vi "Load EEPROM Data FTS Main.vi"(8 "error in (no error)":errorcluster) -> (0 "error out":errorcluster, 3 "EEPROM data":u8[][](array[numeric]) format="%02x")   [LabVIEW 2015]
uses:
  <vilib>/addons/_office/excel.llb/Excel Get Data ([str]).vi
  <vilib>/Utility/NIReport.llb/NI_report.lvclass
  <vilib>/addons/_office/NI_ReportGenerationToolkit.lvlib
  <vilib>/Utility/NIReport.llb/Excel/NI_Excel.lvclass
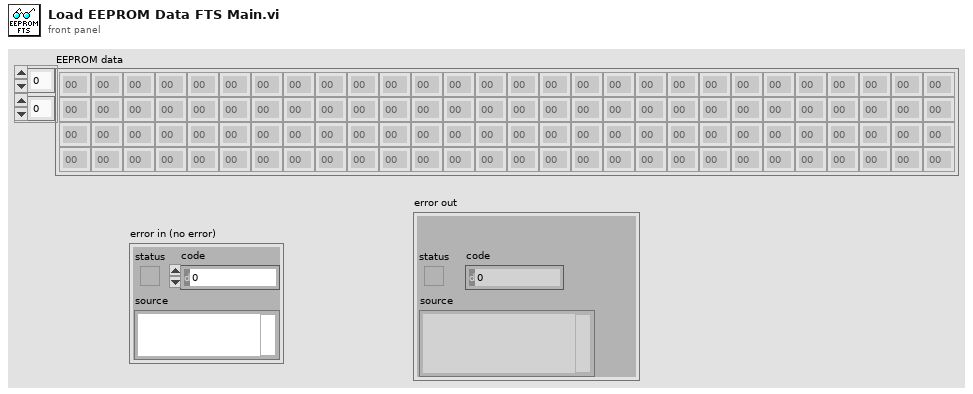
[diagram p1: front panel]
types:
  T1 = enum16{"maximized", "minimized", "normal", "no change"}
  T2 = enum16{"Standard Report", "HTML", "Word", "Excel"}
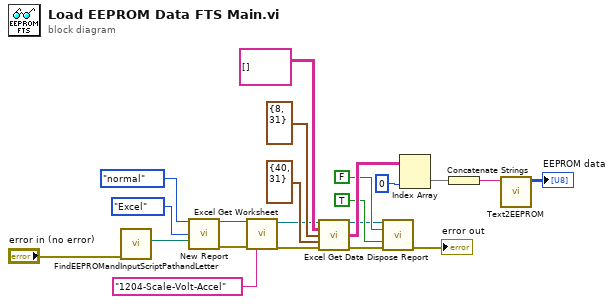
[diagram p0: block diagram]
diagram:
  n1 = call "FindEEPROMandInputScriptPathandLetter.vi"("Error In"="error in (no error)") -> ("Engr Result Path"=w22:path)  [unwired: 6 in, 2 out]
  n2 = call <vilib>:"New Report.vi"("window state (normal)"=T1."normal", "report type"=T2."Excel", "template (empty)"=w22) -> ("report out"=w19:refnum<class "NI_report.lvclass">, "error out"=w18:errorcluster)  [unwired: 11 in]
  n3 = call <vilib>:"Excel Get Worksheet.vi"("report in"=w19, "error in (no error)"=w18, "name (\"\")"="1204-Scale-Volt-Accel" ("name (\"\")")) -> ("report out"=w4:refnum<class "NI_report.lvclass">, "error out"=w6:errorcluster)  [unwired: 11 in]
  n4 = call-poly <vilib>:"Excel Get Data.vi"("report in"=w4, "data type"=string[][] [], "start (-1, -1)"=cluster{"row":i32, "column":i32} {"row"=8, "column"=31}, "end (-1, -1)"=cluster{"row":i32, "column":i32} {"row"=40, "column"=31}, "error in (no error)"=w6) -> ("report out"=w3:refnum<class "NI_report.lvclass">, "data"=w14:string[][], "error out"=w2:errorcluster)  [unwired: 8 in]
  n5 = call-dynamic "Dispose Report.vi"("report in"=w3, "wait until printing completed? (T)"=FALSE, "save changes? (F)"=TRUE, "error in (no error)"=w2) -> ("error out"=→"error out":errorcluster)  [unwired: 11 in]
  n6 = Index Array(array=w14, index (col)=0 ("disabled index (col)")) -> (element=w11:string[])  [unwired: 1 in]
  n7 = Concatenate Strings(w11) -> (w12:string)
  n8 = call "Text2EEPROM.vi"("EEPROM Data"=w12) -> ("EEPROM data"=→"EEPROM data":u8[][])  [unwired: 10 in]
